vi "click counter.vi"() -> ()   [LabVIEW 2013]
panel:
  out "Numeric":dbl
  in  "Boolean":bool
  in  "input":dbl
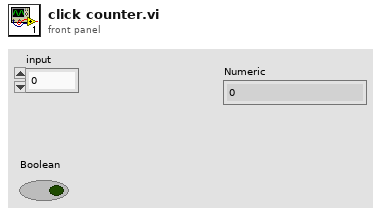
[diagram p1: front panel]
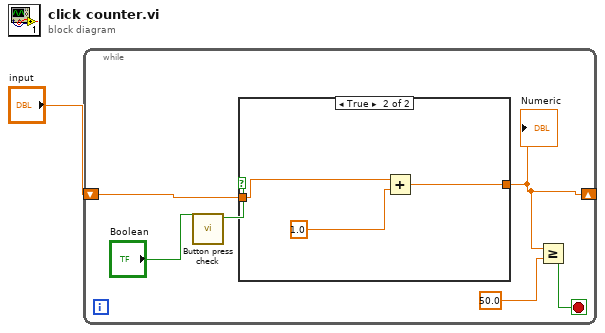
[diagram p0: block diagram]
diagram:
  n1 = while {
    shift-right: [w4] -> _
    shift-left: "input" -> [w7]
    stop <- w2 stop-if-true
    n2 = call "Button press check.vi"("Boolean"="Boolean") -> ("Boolean 2"=w5:bool)  [unwired: 10 in]
    n3 = case shown="True" w5 {
      tunnel: [w8 w10] -> w4
      tunnel: w7 -> [w8 w9]
      frame False {
      }
      frame True {
        n4 = Add(x=w9, y=1.0) -> (x+y=w10:dbl)
      }
    }
    "Numeric" <- w4
    n5 = Greater Or Equal?(x=w4, y=50.0) -> (x >= y?=w2:bool)
  }
